vi "getValue.vi"(8 "error in (no error)":errorcluster, 11 "tBSON_I32 in":refnum<class "tBSON_I32.lvclass">) -> (0 "error out":errorcluster, 2 "Value":i32, 3 "tBSON_I32 out":refnum<class "tBSON_I32.lvclass">)   [LabVIEW 2013, in "BSON.lvlib" / "tBSON_I32.lvclass"]
uses:
  tBSON_I32.lvclass
  tBSON_I32.lvclass/tBSON_I32.ctl
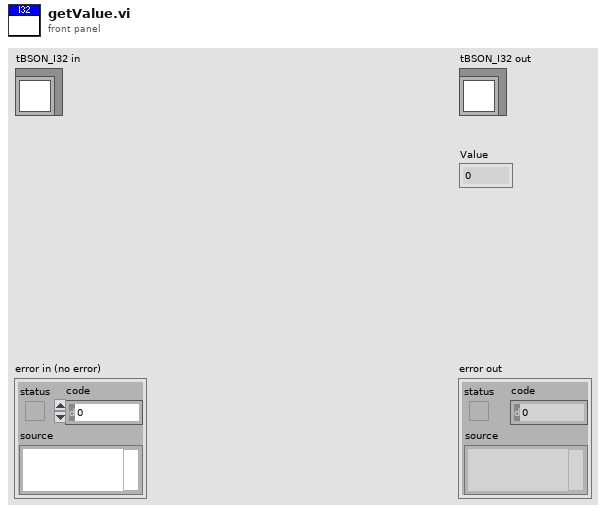
[diagram p1: front panel]
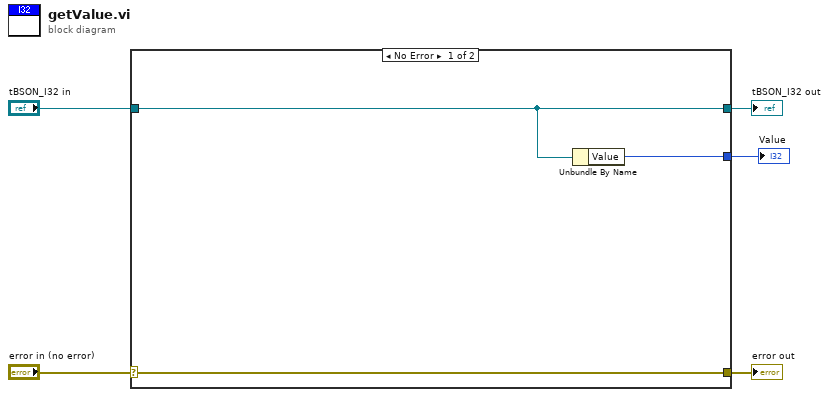
[diagram p0: block diagram]
diagram:
  n1 = case shown="No Error" "error in (no error)" {
    selector: "error in (no error)" -> [w8 w10]
    tunnel: [w8 w10] -> w4
    tunnel: [w7 w9] -> w2
    tunnel: "tBSON_I32 in" -> [w7 w9]
    tunnel: [w6 _] -> w1
    frame No Error {
      n2 = Unbundle By Name(w7) -> ("Value"=w6:i32)
    }
    frame Error {
    }
  }
  "error out" <- w4
  "tBSON_I32 out" <- w2
  "Value" <- w1
